vi "Initialize Instrument.vi"(8 "error in (no error)":errorcluster, 10 "Reset":bool, 11 "VNA-FieldFox in":refnum<class "VNA-FieldFox.lvclass">) -> (0 "error out":errorcluster, 3 "VNA-FieldFox out":refnum<class "VNA-FieldFox.lvclass">)   [LabVIEW 2020, in "VNA-FieldFox.lvclass"]
uses:
  VNA-FieldFox.lvclass
  C:/Sandbox/Git_Sandbox/WiSpry Test Framework source code (LV20)/WiSpry Test Framework/Instruments/Instrument.lvclass
  C:/Sandbox/Git_Sandbox/WiSpry Test Framework source code (LV20)/WiSpry Test Framework/Instruments/Vector Network Analyzer/Vector Network Analyzer.lvclass
  Instrument.lvclass/Instrument.ctl
  Vector Network Analyzer.lvclass/Vector Network Analyzer.ctl
  Instrument.lvclass
  Vector Network Analyzer.lvclass
  <instrlib>/Agilent N99XX Series/Agilent N99XX Series.lvlib
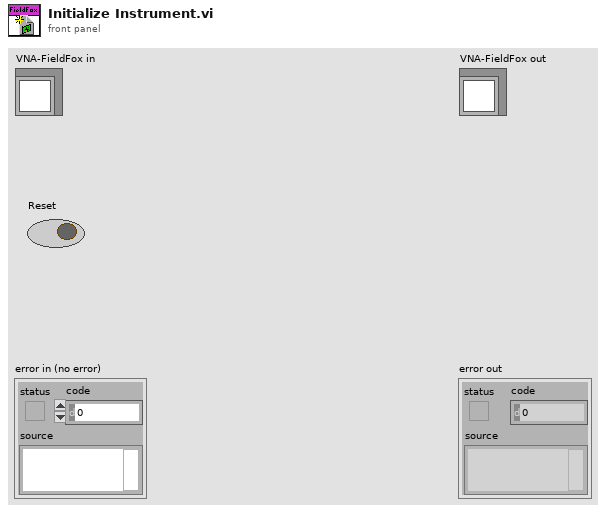
[diagram p1: front panel]
types:
  T1 = typedef "Instrument.lvclass/Interface String Cluster.ctl" = cluster{"Interface":string, "IDN string":string, "Instance":i32}
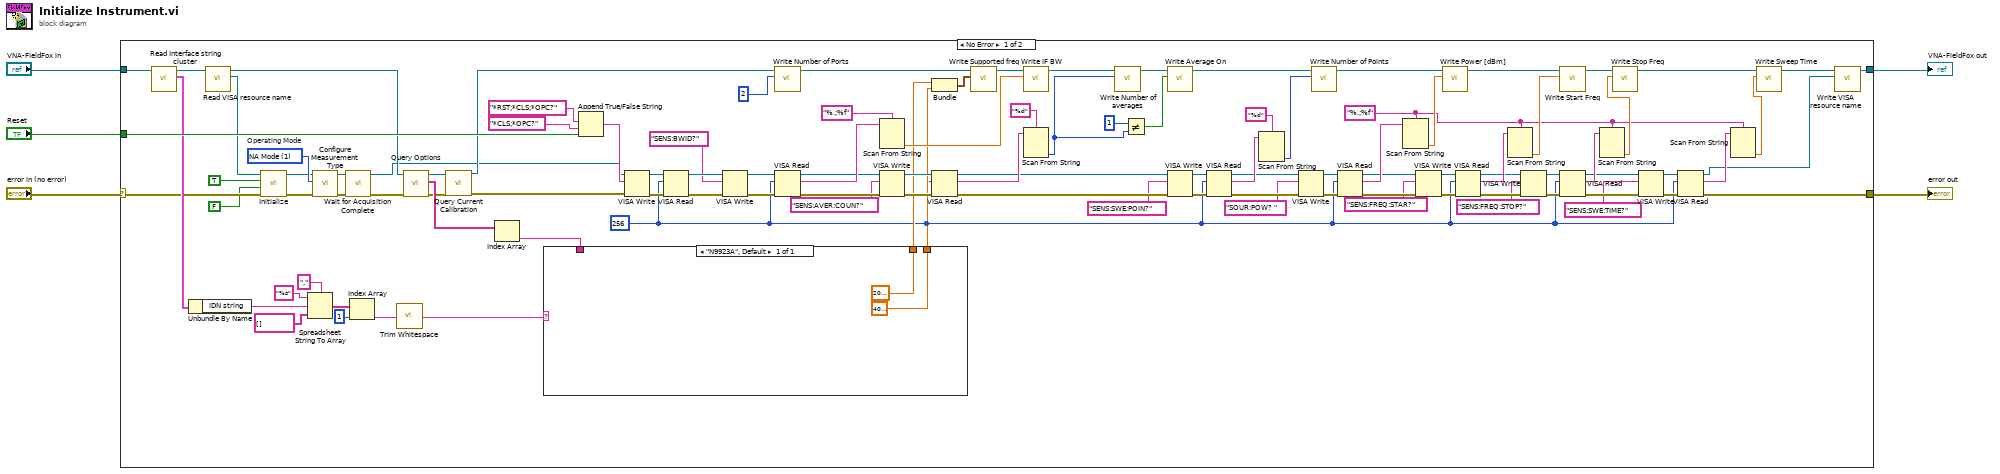
[diagram p0: block diagram]
diagram:
  n1 = case shown="No Error" "error in (no error)" {
    selector: "error in (no error)" -> [w14 w116]
    tunnel: "VNA-FieldFox in" -> [w39 w117]
    tunnel: [w27 w116] -> w2
    tunnel: [w91 w117] -> w1
    tunnel: "Reset" -> [w43 _]
    frame No Error {
      w16 = 1 items=["CAT Mode", "NA Mode", "SA Mode", "PM Mode", "VVM Mode"]  # Operating Mode
      w45 = "%.;%f" ("format string")
      w24 = u32 256 ("byte count")
      n2 = call "Read Interface string cluster.vi"("Instrument in"=w39) -> ("Interface sting cluster"=w42:T1, "Instrument out"=w38:refnum<class "VNA-FieldFox.lvclass">)  [unwired: 9 in]
      n3 = Unbundle By Name(w42) -> ("IDN string"=w35:string)
      n4 = call "Read VISA resource name.vi"("Instrument in"=w38) -> ("VISA resource name"=w13:refnum<visa-resource-name>, "Instrument out"=w37:refnum<class "VNA-FieldFox.lvclass">)  [unwired: 9 in]
      n5 = call <instrlib>:"Initialize.vi"("error in (no error)"=w14, "Reset (True)"=FALSE, "ID Query (True)"=TRUE, "VISA resource name"=w13) -> ("error out"=w10:errorcluster, "VISA resource name out"=w9:refnum<visa-resource-name>)  [unwired: 6 in]
      n6 = Spreadsheet String To Array(delimiter (Tab)=",", format string="%s", spreadsheet string=w35, array type (2D Dbl)=string[] []) -> (array=w36:string[])
      n7 = call <instrlib>:"Configure Measurement Type.vi"("error in (no error)"=w10, "Operating Mode (0: CAT Mode)"=w16, "VISA resource name"=w9) -> ("error out"=w8:errorcluster, "VISA resource name out"=w15:refnum<visa-resource-name>)  [unwired: 7 out]
      n8 = call <instrlib>:"Wait for Acquisition Complete.vi"("error in (no error)"=w8, "VISA resource name"=w15) -> ("error out"=w7:errorcluster, "VISA resource name out"=w6:refnum<visa-resource-name>)  [unwired: 1 in, 7 out]
      n9 = Index Array(array=w36, index=1) -> (element=w29:string)
      n10 = call <vilib>:"Trim Whitespace.vi"("string"=w29) -> ("trimmed string"=w28:string)  [unwired: 1 in]
      n11 = call-dynamic "Query Options.vi"("error in (no error)"=w7, "Instrument in"=w37) -> ("error out"=w21:errorcluster, "Options"=w30:string[], "Instrument out"=w23:refnum<class "VNA-FieldFox.lvclass">)  [unwired: 7 in]
      n12 = call-dynamic "Query Current Calibration.vi"("error in (no error)"=w21, "Vector Network Analyzer in"=w23) -> ("error out"=w20:errorcluster, "Vector Network Analyzer out"=w22:refnum<class "VNA-FieldFox.lvclass">)  [unwired: 8 in]
      n13 = Index Array(array=w30) -> (element=w25:string)  [unwired: 1 in]
      n14 = case shown="\"N9923A\", Default" w28 {
        tunnel: [4000000000.0] -> w32
        tunnel: [2000000.0] -> w31
        tunnel: w25 -> [_]
        frame "N9923A", Default {
        }
      }
      n15 = Append True/False String(1:w43, 2:"*CLS;*OPC?" ("false string"), 3:"*RST;*CLS;*OPC?" ("Default Setup String")) -> (0:w111:string)  [unwired: 1 in]
      n16 = VISA Write(VISA resource name=w6, write buffer=w111, error in (no error)=w20) -> (VISA resource name out=w109:refnum<visa-resource-name>, error out=w110:errorcluster)  [unwired: 1 out]
      n17 = VISA Read(VISA resource name=w109, byte count=w24, error in (no error)=w110) -> (VISA resource name out=w98:refnum<visa-resource-name>, error out=w99:errorcluster)  [unwired: 2 out]
      n18 = VISA Write(VISA resource name=w98, write buffer="SENS:BWID?", error in (no error)=w99) -> (VISA resource name out=w100:refnum<visa-resource-name>, error out=w96:errorcluster)  [unwired: 1 out]
      n19 = call "Write Number of Ports.vi"("Number of Ports"=2, "Vector Network Analyzer in"=w22) -> ("Vector Network Analyzer out"=w108:refnum<class "VNA-FieldFox.lvclass">)  [unwired: 9 in]
      n20 = VISA Read(VISA resource name=w100, byte count=w24, error in (no error)=w96) -> (VISA resource name out=w89:refnum<visa-resource-name>, read buffer=w94:string, error out=w88:errorcluster)  [unwired: 1 out]
      n21 = Scan From String(format string="%.;%f", input string=w94) -> (output 1=w93:dbl)  [unwired: 3 in, 3 out]
      n22 = VISA Write(VISA resource name=w89, write buffer="SENS:AVER:COUN?", error in (no error)=w88) -> (VISA resource name out=w86:refnum<visa-resource-name>, error out=w90:errorcluster)  [unwired: 1 out]
      n23 = Bundle(w31, w32) -> (w107:cluster{dbl, dbl})  [unwired: 1 in]
      n24 = VISA Read(VISA resource name=w86, byte count=w24, error in (no error)=w90) -> (VISA resource name out=w83:refnum<visa-resource-name>, read buffer=w85:string, error out=w82:errorcluster)  [unwired: 1 out]
      n25 = call "Write Supported freq.vi"("Supported freq"=w107, "Vector Network Analyzer in"=w108) -> ("Vector Network Analyzer out"=w92:refnum<class "VNA-FieldFox.lvclass">)  [unwired: 9 in]
      n26 = call "Write IF BW.vi"("IF BW"=w93, "Vector Network Analyzer in"=w92) -> ("Vector Network Analyzer out"=w106:refnum<class "VNA-FieldFox.lvclass">)  [unwired: 9 in]
      n27 = Scan From String(format string="%d", input string=w85) -> (output 1=w18:i32)  [unwired: 3 in, 3 out]
      n28 = call "Write Number of averages.vi"("Number of averages"=w18, "Vector Network Analyzer in"=w106) -> ("Vector Network Analyzer out"=w105:refnum<class "VNA-FieldFox.lvclass">)  [unwired: 9 in]
      n29 = Not Equal?(x=1, y=w18) -> (x != y?=w81:bool)
      n30 = call "Write Average On.vi"("Average On"=w81, "Vector Network Analyzer in"=w105) -> ("Vector Network Analyzer out"=w104:refnum<class "VNA-FieldFox.lvclass">)  [unwired: 9 in]
      n31 = VISA Write(VISA resource name=w83, write buffer="SENS:SWE:POIN?", error in (no error)=w82) -> (VISA resource name out=w79:refnum<visa-resource-name>, error out=w80:errorcluster)  [unwired: 1 out]
      n32 = VISA Read(VISA resource name=w79, byte count=w24, error in (no error)=w80) -> (VISA resource name out=w72:refnum<visa-resource-name>, read buffer=w76:string, error out=w71:errorcluster)  [unwired: 1 out]
      n33 = Scan From String(format string="%d", input string=w76) -> (output 1=w75:i32)  [unwired: 3 in, 3 out]
      n34 = VISA Write(VISA resource name=w72, write buffer="SOUR:POW? ", error in (no error)=w71) -> (VISA resource name out=w74:refnum<visa-resource-name>, error out=w73:errorcluster)  [unwired: 1 out]
      n35 = call "Write Number of Points.vi"("Number of Points"=w75, "Vector Network Analyzer in"=w104) -> ("Vector Network Analyzer out"=w103:refnum<class "VNA-FieldFox.lvclass">)  [unwired: 9 in]
      n36 = VISA Read(VISA resource name=w74, byte count=w24, error in (no error)=w73) -> (VISA resource name out=w65:refnum<visa-resource-name>, read buffer=w69:string, error out=w64:errorcluster)  [unwired: 1 out]
      n37 = Scan From String(format string=w45, input string=w69) -> (output 1=w68:dbl)  [unwired: 3 in, 3 out]
      n38 = VISA Write(VISA resource name=w65, write buffer="SENS:FREQ:STAR?", error in (no error)=w64) -> (VISA resource name out=w66:refnum<visa-resource-name>, error out=w67:errorcluster)  [unwired: 1 out]
      n39 = call "Write Power [dBm].vi"("Power [dBm]"=w68, "Vector Network Analyzer in"=w103) -> ("Vector Network Analyzer out"=w102:refnum<class "VNA-FieldFox.lvclass">)  [unwired: 9 in]
      n40 = VISA Read(VISA resource name=w66, byte count=w24, error in (no error)=w67) -> (VISA resource name out=w59:refnum<visa-resource-name>, read buffer=w62:string, error out=w58:errorcluster)  [unwired: 1 out]
      n41 = Scan From String(format string=w45, input string=w62) -> (output 1=w61:dbl)  [unwired: 3 in, 3 out]
      n42 = VISA Write(VISA resource name=w59, write buffer="SENS:FREQ:STOP?", error in (no error)=w58) -> (VISA resource name out=w60:refnum<visa-resource-name>, error out=w56:errorcluster)  [unwired: 1 out]
      n43 = call "Write Start Freq.vi"("Start Freq"=w61, "Vector Network Analyzer in"=w102) -> ("Vector Network Analyzer out"=w101:refnum<class "VNA-FieldFox.lvclass">)  [unwired: 9 in]
      n44 = VISA Read(VISA resource name=w60, byte count=w24, error in (no error)=w56) -> (VISA resource name out=w51:refnum<visa-resource-name>, read buffer=w54:string, error out=w50:errorcluster)  [unwired: 1 out]
      n45 = Scan From String(format string=w45, input string=w54) -> (output 1=w55:dbl)  [unwired: 3 in, 3 out]
      n46 = call "Write Stop Freq.vi"("Stop Freq"=w55, "Vector Network Analyzer in"=w101) -> ("Vector Network Analyzer out"=w48:refnum<class "VNA-FieldFox.lvclass">)  [unwired: 9 in]
      n47 = VISA Write(VISA resource name=w51, write buffer="SENS:SWE:TIME?", error in (no error)=w50) -> (VISA resource name out=w52:refnum<visa-resource-name>, error out=w53:errorcluster)  [unwired: 1 out]
      n48 = VISA Read(VISA resource name=w52, byte count=w24, error in (no error)=w53) -> (VISA resource name out=w26:refnum<visa-resource-name>, read buffer=w46:string, error out=w27:errorcluster)  [unwired: 1 out]
      n49 = Scan From String(format string=w45, input string=w46) -> (output 1=w44:dbl)  [unwired: 3 in, 3 out]
      n50 = call "Write Sweep Time.vi"("Sweep Time"=w44, "Vector Network Analyzer in"=w48) -> ("Vector Network Analyzer out"=w47:refnum<class "VNA-FieldFox.lvclass">)  [unwired: 9 in]
      n51 = call "Write VISA resource name.vi"("VISA resource name"=w26, "Instrument in"=w47) -> ("Instrument out"=w91:refnum<class "VNA-FieldFox.lvclass">)  [unwired: 9 in]
    }
    frame Error {
    }
  }
  "error out" <- w2
  "VNA-FieldFox out" <- w1
